vi "cinitel_stabilizace.vi"() -> ()   [LabVIEW 2024]
uses:
  <vilib>/Analysis/baseanly.llb/Mean (DBL).vi
  <instrlib>/EFmeter/EFmeter.lvlib
  <vilib>/Analysis/NI_AALBase.lvlib
  <instrlib>/Zatez Kopper/Zatez Kopper.lvlib
panel:
  in  "Typ zateze":u16(ring) items=["Manualni", "BK 8542B", "Zatez Kopper"]
  in  "VISA EFmeter":refnum<visa-resource-name>
  out "R_out":dbl
  in  "file path (use dialog)":path
  in  "Prodleva mezi vzorky":u32
  out "Aktualni zatez":dbl=2.5
  in  "velikost kroku":dbl
  in  "start":dbl
  in  "Prumerovani":bool
  in  "Vzorku na krokù":u16 max=100 step=1
  out "XY Graph 2":cluster{"X":dbl[], "Y":dbl[]}[](graph)
  in  "Pocet kroku":i32
  in  "Clear":bool
  in  "Uložit data":bool
  in  "Start":bool
  in  "VISA  zatez":refnum<visa-resource-name>
  in  "stop":bool
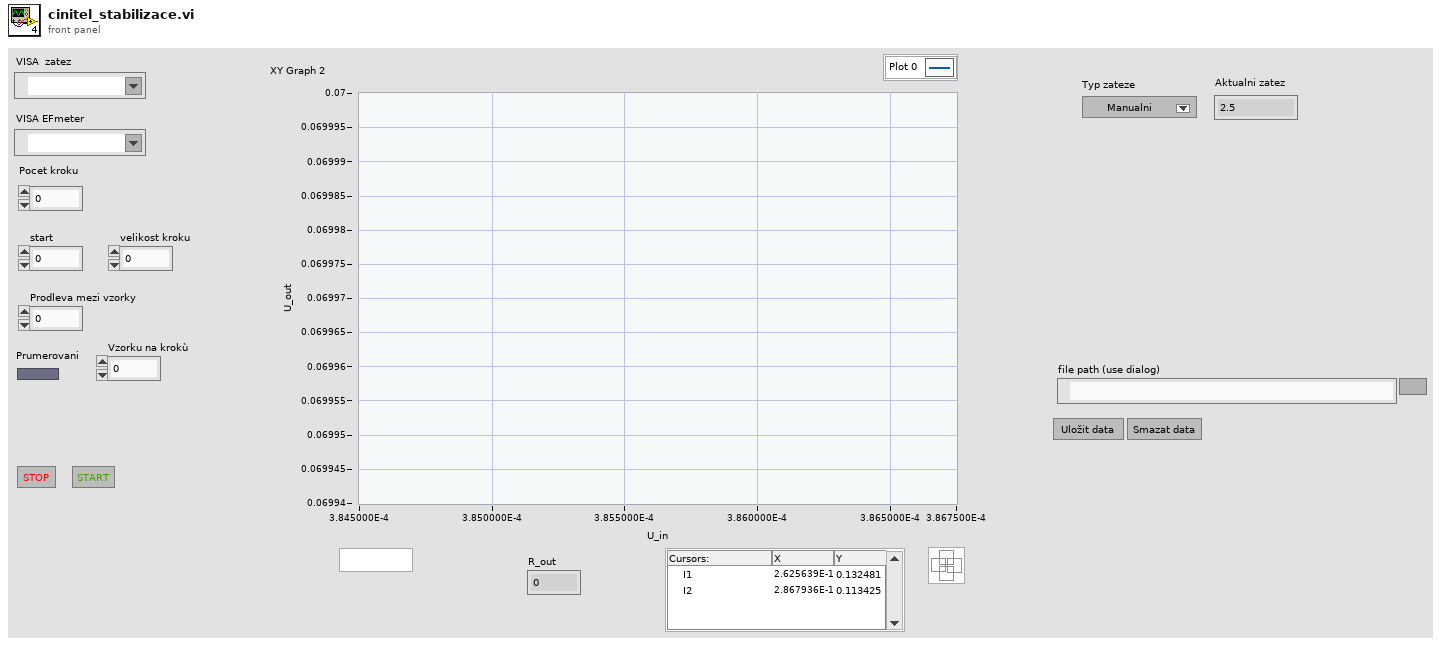
[diagram p1: front panel]
types:
  T1 = enum16{"init", "wait", "graph", "meas", "change_load", "init_measurment", "save", "clear"}
  T2 = typedef "LVCursorListTypeDef.ctl" = cluster{"Name":string, "Color":u32, "Style":u8, "Point Style":u8, "Name Visible":bool, "Allow Drag":bool, "Cursor Mode":u32, "Plot":i32, "Index":i32, "Position":cluster{"X":dbl, "Y":dbl}, "X Scale":u32, "Y Scale":u32, "Watch Plots":i32[], "Watch All Plots":bool, "Plot Area":i32, "Label Offset":cluster{"X":dbl, "Y":dbl}}[]
  T3 = cluster{"Name":string, "Color":u32, "Style":u8, "Point Style":u8, "Name Visible":bool, "Allow Drag":bool, "Cursor Mode":u32, "Plot":i32, "Index":i32, "Position":cluster{"X":dbl, "Y":dbl}, "X Scale":u32, "Y Scale":u32, "Watch Plots":i32[], "Watch All Plots":bool, "Plot Area":i32, "Label Offset":cluster{"X":dbl, "Y":dbl}}
  T4 = enum16{"open", "replace", "create", "open or create", "replace or create", "replace or create with confirmation"}
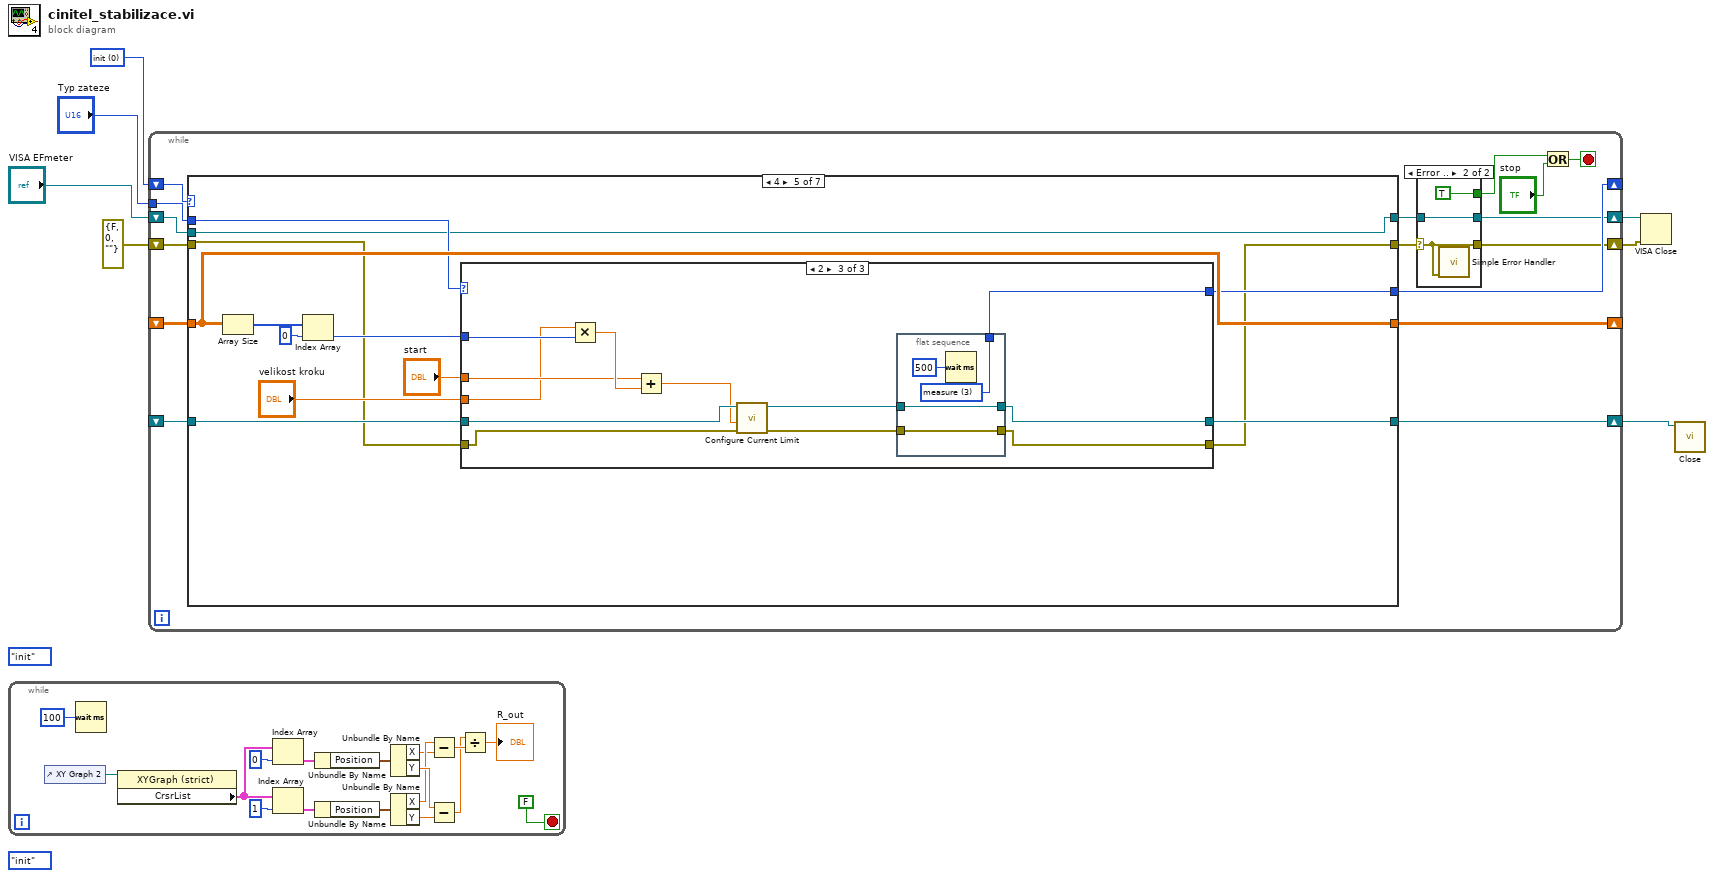
[diagram p0: block diagram]
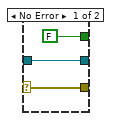
[diagram p2: hidden frame]
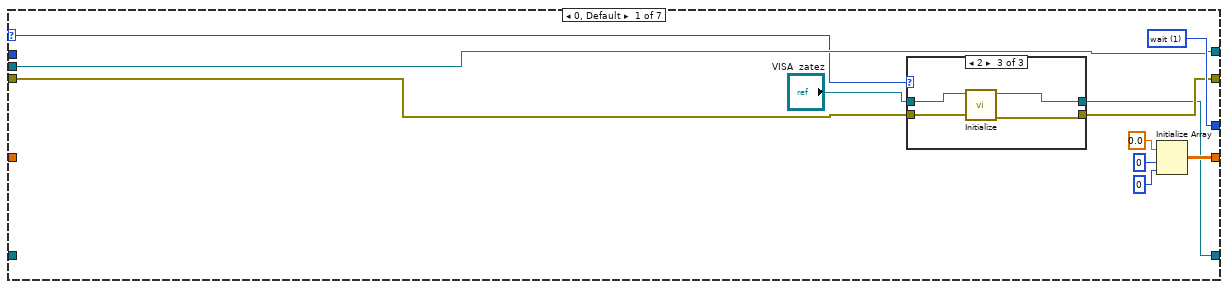
[diagram p3: hidden frame]
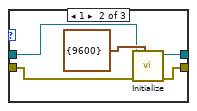
[diagram p5: hidden frame]
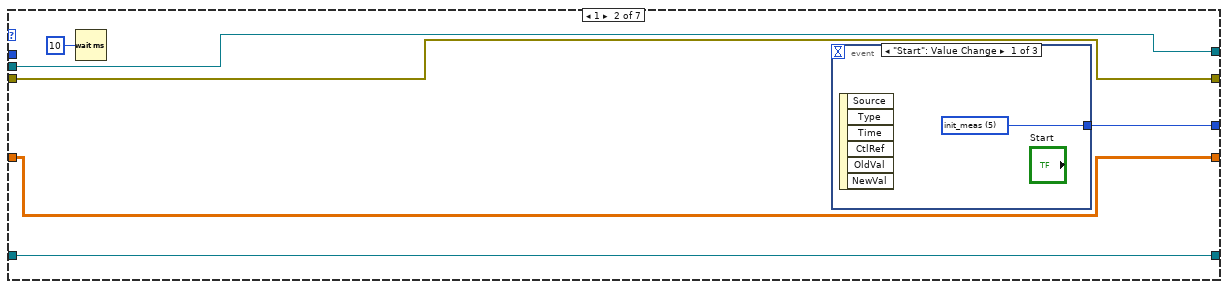
[diagram p6: hidden frame]
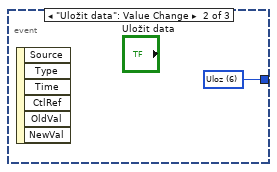
[diagram p7: hidden frame]
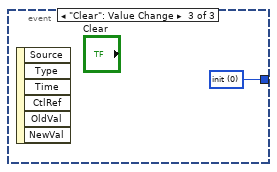
[diagram p8: hidden frame]
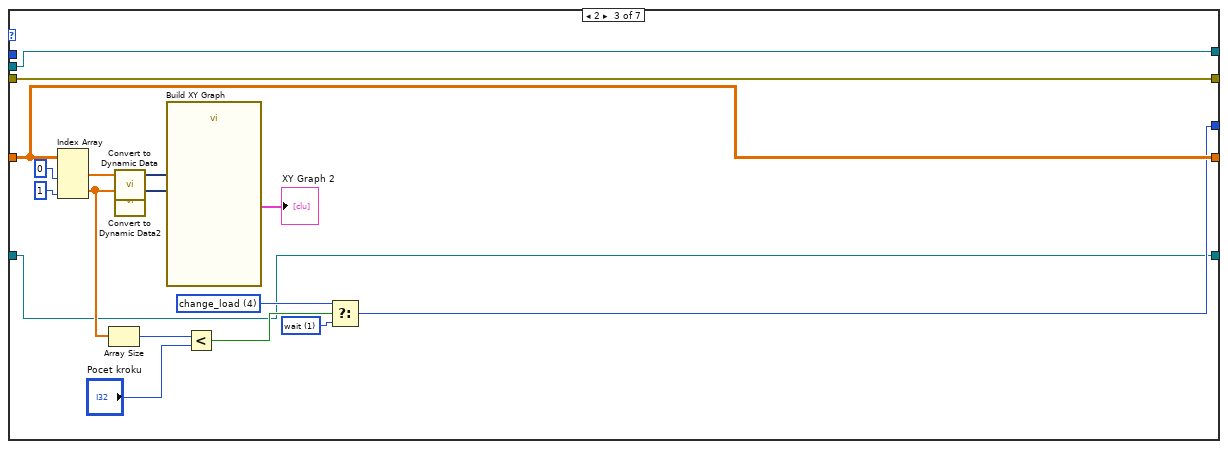
[diagram p9: hidden frame]
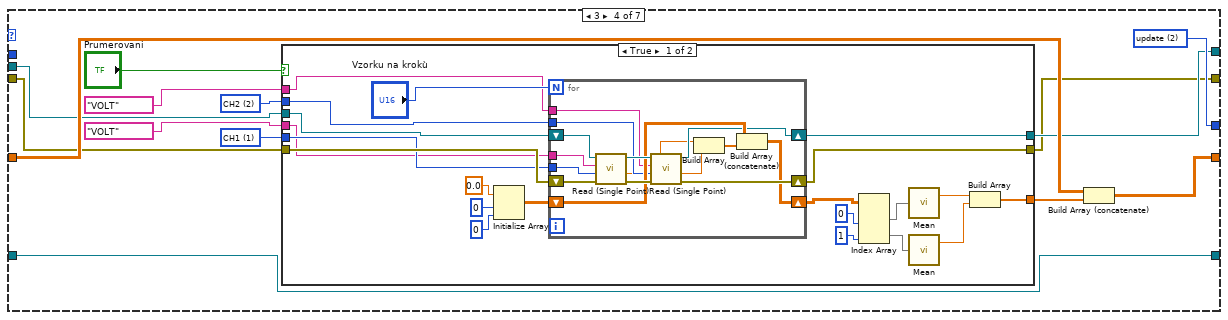
[diagram p10: hidden frame]
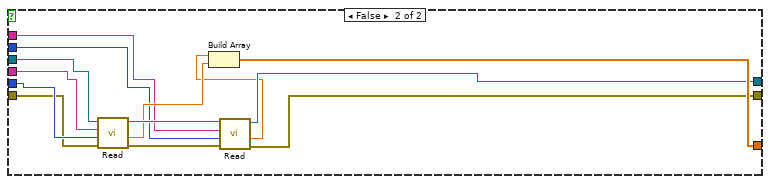
[diagram p11: hidden frame]
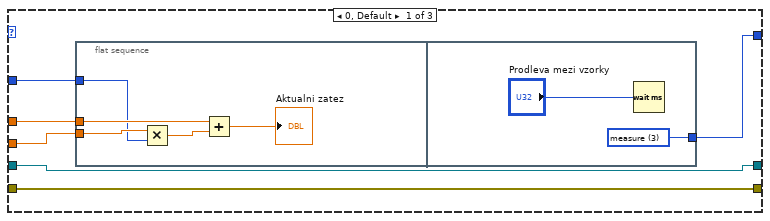
[diagram p12: hidden frame]
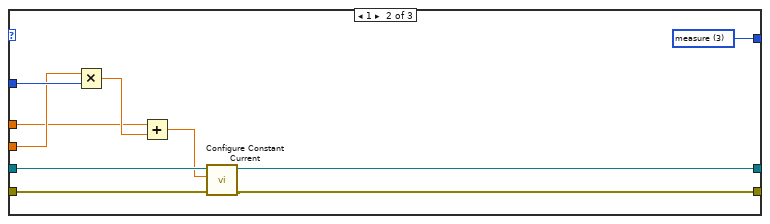
[diagram p13: hidden frame]
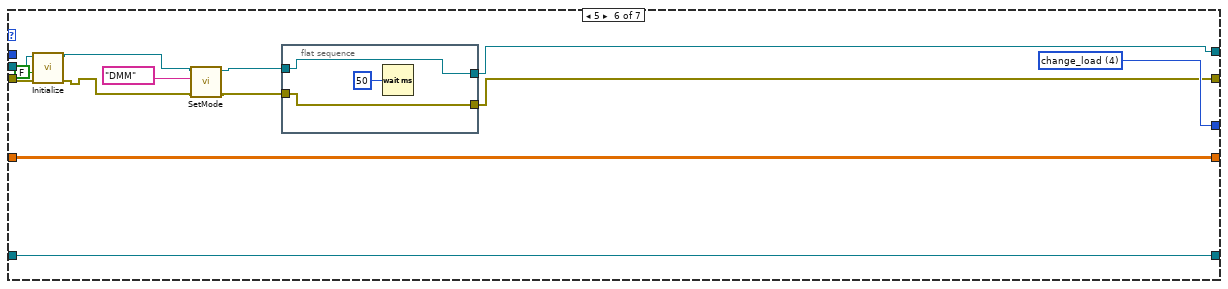
[diagram p14: hidden frame]
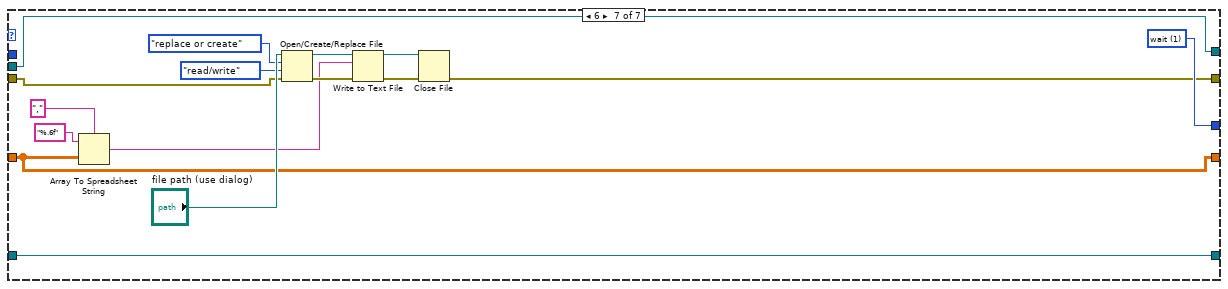
[diagram p15: hidden frame]
diagram:
  (unwired) T1."init"
  (unwired) T1."init"
  w7 = u16 0 items=["init", "wait", "update", "measure", "change_load", "init_meas", "Uloz", "clear"]
  n1 = while {
    stop <- FALSE stop-if-true
    n2 = control-ref of="XY Graph 2"() -> (w22:refnum<vi>)
    n3 = Wait (ms)(milliseconds to wait=u32 100) -> ()  [unwired: 1 out]
    n4 = property class="XYGraph (strict)"(reference=w22) -> ("CrsrList"=w17:T2)  [unwired: 1 in, 2 out]
    n5 = Index Array(array=w17, index=0) -> (element=w23:T3)
    n6 = Index Array(array=w17, index=1) -> (element=w19:T3)
    n7 = Unbundle By Name(w23) -> ("Position"=w24:cluster{"X":dbl, "Y":dbl})
    n8 = Unbundle By Name(w19) -> ("Position"=w20:cluster{"X":dbl, "Y":dbl})
    n9 = Unbundle By Name(w24) -> ("X"=w8:dbl, "Y"=w15:dbl)
    n10 = Unbundle By Name(w20) -> ("X"=w9:dbl, "Y"=w16:dbl)
    n11 = Subtract(x=w9, y=w8) -> (x-y=w11:dbl)
    n12 = Subtract(x=w15, y=w16) -> (x-y=w10:dbl)
    n13 = Divide(x=w10, y=w11) -> (x/y=→"R_out":dbl)
  }
  n14 = while {
    shift-right: [w40] -> _
    shift-left: _ -> [w39]
    shift-right: [w35] -> _
    shift-left: w7 -> [w38]
    shift-right: [w32] -> w4
    shift-left: "VISA EFmeter" -> [w37]
    shift-right: [w25] -> w3
    shift-left: errorcluster {"status"=FALSE, "code"=0, "source"=""} ("error in (no error)") -> [w36]
    tunnel: "Typ zateze" -> [w28]
    shift-right: [w27] -> w1
    shift-left: _ -> [w26]
    stop <- w30 stop-if-true
    n15 = case shown="4" w38 {
      selector: w38 -> [w51 _ _ _ _ _ _]
      tunnel: [w55 w73 w86 w107 w170 w222 w236] -> w40
      tunnel: w39 -> [_ w73 w86 w108 w170 w222 w236]
      tunnel: [w54 w74 w85 w105 w168 w221 w234] -> w35
      tunnel: [w49 w71 w79 w97 w158 w219 w230] -> w34
      tunnel: [w52 w72 w80 w98 w167 w220 w241] -> w33
      tunnel: w37 -> [w52 w72 w80 w104 w167 w217 w241]
      tunnel: w36 -> [w50 w71 w79 w103 w159 w216 w237]
      tunnel: w28 -> [_ _ _ _ w169 _ _]
      tunnel: [w48 w69 w78 w95 w165 w218 w226] -> w27
      tunnel: w26 -> [_ w69 w78 w95 w166 w218 w226]
      frame 0, Default {
        w54 = u16 1 items=["init", "wait", "update", "measure"]
        n16 = case shown="2" w51 {
          tunnel: w50 -> [w59 w63 w68]
          tunnel: [w59 w62 w65] -> w49
          tunnel: [w58 w61 w66] -> w48
          tunnel: "VISA  zatez" -> [w58 w60 w67]
          frame 0, Default {
          }
          frame 1 {
            n17 = call <instrlib>:"Initialize.vi"("Serial Configuration"=cluster{"Baud Rate":u32} {"Baud Rate"=9600}, "error in (no error)"=w63, "VISA resource name"=w60) -> ("error out"=w62:errorcluster, "VISA resource name out"=w61:refnum<visa-resource-name>)  [unwired: 7 in]
          }
          frame 2 {
            n18 = call <instrlib>:"Initialize.vi"("error in (no error)"=w68, "VISA resource name"=w67) -> ("error out"=w65:errorcluster, "VISA resource name out"=w66:refnum<visa-resource-name>)  [unwired: 8 in]
          }
        }
        n19 = Initialize Array(0.0 ("element"), 0 ("dimension size"), 0 ("dimension size")) -> (w55:dbl[][])
      }
      frame 1 {
        n20 = Wait (ms)(milliseconds to wait=u32 10) -> ()  [unwired: 1 out]
        n21 = event shown="[0] \"Start\": Value Change" {
          selector: _ -> [_ _ _]
          dyn-events: _ -> [_ _ _]
          timeout: _ -> [_ _ _]
          tunnel: [w75 w76 w77] -> w74
          event "Start": Value Change {
            w75 = u16 5 items=["init", "wait", "update", "measure", "change_load", "init_meas"]
            n22 = event-data() -> ()  [unwired: 1 in, 6 out]
          }
          event "Uložit data": Value Change {
            w76 = u16 6 items=["init", "wait", "update", "measure", "change_load", "init_meas", "Uloz"]
            n23 = event-data() -> ()  [unwired: 1 in, 6 out]
          }
          event "Clear": Value Change {
            w77 = u16 0 items=["init", "wait", "update", "measure", "change_load", "init_meas", "Uloz", "clear"]
            n24 = event-data() -> ()  [unwired: 1 in, 6 out]
          }
        }
      }
      frame 2 {
        w81 = u16 4 items=["init", "wait", "update", "measure", "change_load", "init_meas"]
        w87 = u16 1 items=["init", "wait", "update", "measure"]
        n25 = Index Array(array=w86, index (col) #1=0 ("index (row)"), index (col) #2=1 ("index (row)")) -> (element #1=w94:dbl[], element #2=w89:dbl[])  [unwired: 2 in]
        n26 = Array Size(array=w89) -> (size(s)=w91:i32)
        n27 = call "Convert to Dynamic Data"("Array"=w94) -> ("Dynamic Data Type"=w93:dynamicdata)  [unwired: 3 in]
        n28 = call "Convert to Dynamic Data2"("Array"=w89) -> ("Dynamic Data Type"=w92:dynamicdata)  [unwired: 3 in]
        n29 = call "Build XY Graph"("Y Input"=w92, "X Input"=w93) -> ("XY Graph"=→"XY Graph 2":cluster{"X":dbl[], "Y":dbl[]}[])  [unwired: 8 in, 1 out]
        n30 = Less?(x=w91, y="Pocet kroku") -> (x < y?=w90:bool)
        n31 = Select(t=w81, s=w90, f=w87) -> (s? t:f=w85:u16)
      }
      frame 3 {
        w99 = u16 2 items=["CH2"=2, "CH1"=1] ("Ring")
        w102 = u16 1 items=["CH2"=2, "CH1"=1] ("Ring")
        w105 = u16 2 items=["init", "wait", "update", "measure"]
        n32 = case shown="True" "Prumerovani" {
          tunnel: [w111 w157] -> w106
          tunnel: w104 -> [w124 w156]
          tunnel: w103 -> [w123 w153]
          tunnel: w102 -> [w122 w154]
          tunnel: "VOLT" ("Combo Box") -> [w121 w155]
          tunnel: "VOLT" ("Combo Box") -> [w120 w149]
          tunnel: w99 -> [w119 w148]
          tunnel: [w110 w147] -> w98
          tunnel: [w109 w146] -> w97
          frame True {
            n33 = Initialize Array(0.0 ("element"), 0 ("dimension size"), 0 ("dimension size")) -> (w125:dbl[][])
            n34 = for {
              N: "Vzorku na krokù" -> [_]
              shift-right: [w140] -> w110
              shift-left: w124 -> [w141]
              shift-right: [w138] -> w109
              shift-left: w123 -> [w139]
              tunnel: w122 -> [w137]
              tunnel: w121 -> [w136]
              tunnel: w120 -> [w135]
              tunnel: w119 -> [w134]
              shift-right: [w133] -> w118
              shift-left: w125 -> [w142]
              n35 = call <instrlib>:"Read (Single Point).vi"("error in (no error)"=w139, "Ring"=w137, "Combo Box"=w136, "VISA resource name"=w141) -> ("error out"=w143:errorcluster, "Measurement"=w131:dbl, "VISA resource name out"=w144:refnum<visa-resource-name>)  [unwired: 5 in]
              n36 = call <instrlib>:"Read (Single Point).vi"("error in (no error)"=w143, "Ring"=w134, "Combo Box"=w135, "VISA resource name"=w144) -> ("error out"=w138:errorcluster, "Measurement"=w132:dbl, "VISA resource name out"=w140:refnum<visa-resource-name>)  [unwired: 5 in]
              n37 = Build Array(w131, w132) -> (w130:dbl[])
              n38 = Build Array (concatenate)(w142, w130) -> (w133:dbl[][])
            }
            n39 = Index Array(array=w118, index (col) #1=0 ("disabled index (col)"), index (col) #2=1 ("index (col)")) -> (element #1=w117:dbl[], element #2=w116:dbl[])  [unwired: 2 in]
            n40 = call-poly <vilib>:"Mean.vi"("X"=w117) -> ("mean"=w113:dbl)  [unwired: 1 out]
            n41 = call-poly <vilib>:"Mean.vi"("X"=w116) -> ("mean"=w112:dbl)  [unwired: 1 out]
            n42 = Build Array(w113, w112) -> (w111:dbl[])
          }
          frame False {
            n43 = call-poly <instrlib>:"Read.vi"("error in (no error)"=w153, "Ring"=w154, "Combo Box"=w155, "VISA resource name"=w156) -> ("error out"=w151:errorcluster, "Measurement"=w150:dbl, "VISA resource name out"=w152:refnum<visa-resource-name>)  [unwired: 5 in]
            n44 = call-poly <instrlib>:"Read.vi"("error in (no error)"=w151, "Ring"=w148, "Combo Box"=w149, "VISA resource name"=w152) -> ("error out"=w146:errorcluster, "Measurement"=w145:dbl, "VISA resource name out"=w147:refnum<visa-resource-name>)  [unwired: 5 in]
            n45 = Build Array(w145, w150) -> (w157:dbl[])
          }
        }
        n46 = Build Array (concatenate)(w108, w106) -> (w107:dbl[][])
      }
      frame 4 {
        n47 = Array Size(array=w170) -> (size(s)=w160:i32[])
        n48 = Index Array(array=w160, index=0) -> (element=w162:i32)
        n49 = case shown="2" w169 {
          tunnel: [w176 w193 w194] -> w168
          tunnel: w166 -> [w175 w192 w200]
          tunnel: [w175 w191 w195] -> w165
          tunnel: "velikost kroku" -> [w174 w189 w202]
          tunnel: "start" -> [w173 w187 w203]
          tunnel: w162 -> [w172 w190 w204]
          tunnel: w159 -> [w171 w185 w201]
          tunnel: [w171 w184 w197] -> w158
          frame 0, Default {
            n50 = flat-sequence {
              tunnel: w174 -> [w179]
              tunnel: w173 -> [w178]
              tunnel: w172 -> [w177]
              tunnel: [w182] -> w176
              frame #0 {
                n51 = Multiply(x=w179, y=w177) -> (x*y=w181:dbl)
                n52 = Add(x=w178, y=w181) -> (x+y=→"Aktualni zatez":dbl)
              }
              frame #1 {
                w182 = u16 3 items=["init", "wait", "update", "measure", "change_load", "init_meas"]
                n53 = Wait (ms)(milliseconds to wait="Prodleva mezi vzorky") -> ()  [unwired: 1 out]
              }
            }
          }
          frame 1 {
            w193 = u16 3 items=["init", "wait", "update", "measure", "change_load", "init_meas"]
            n54 = Multiply(x=w189, y=w190) -> (x*y=w188:dbl)
            n55 = Add(x=w187, y=w188) -> (x+y=w186:dbl)
            n56 = call "Configure Constant Current.vi"("error in (no error)"=w185, "CC Current (0)"=w186, "VISA resource name"=w192) -> ("error out"=w184:errorcluster, "VISA resource name out"=w191:refnum<visa-resource-name>)  [unwired: 7 in]
          }
          frame 2 {
            n57 = Multiply(x=w202, y=w204) -> (x*y=w205:dbl)
            n58 = Add(x=w203, y=w205) -> (x+y=w199:dbl)
            n59 = call <instrlib>:"Configure Current Limit.vi"("error in (no error)"=w201, "Current Limit (0.0 A)"=w199, "VISA resource name"=w200) -> ("error out"=w198:errorcluster, "VISA resource name out"=w196:refnum<visa-resource-name>)  [unwired: 7 in]
            n60 = flat-sequence {
              tunnel: w198 -> [w209]
              tunnel: [w209] -> w197
              tunnel: [w208] -> w195
              tunnel: w196 -> [w208]
              tunnel: [w207] -> w194
              frame #0 {
                w207 = u16 3 items=["init", "wait", "update", "measure", "change_load", "init_meas", "Uloz", "clear"]
                n61 = Wait (ms)(milliseconds to wait=u32 500) -> ()  [unwired: 1 out]
              }
            }
          }
        }
      }
      frame 5 {
        w221 = u16 4 items=["init", "wait", "update", "measure", "change_load", "init_meas"]
        n62 = call <instrlib>:"Initialize.vi"("error in (no error)"=w216, "Reset (True)"=FALSE, "VISA resource name"=w217) -> ("error out"=w213:errorcluster, "VISA resource name out"=w214:refnum<visa-resource-name>)  [unwired: 7 in]
        n63 = call <instrlib>:"SetMode.vi"("error in (no error)"=w213, "Combo Box"="DMM", "VISA resource name"=w214) -> ("error out"=w212:errorcluster, "VISA resource name out"=w211:refnum<visa-resource-name>)  [unwired: 7 in]
        n64 = flat-sequence {
          tunnel: [w224] -> w220
          tunnel: w211 -> [w224]
          tunnel: w212 -> [w223]
          tunnel: [w223] -> w219
          frame #0 {
            n65 = Wait (ms)(milliseconds to wait=u32 50) -> ()  [unwired: 1 out]
          }
        }
      }
      frame 6 {
        w234 = u16 1 items=["init", "wait", "update", "measure", "change_load", "init_meas"]
        n66 = Array To Spreadsheet String(delimiter (Tab)=",", array=w236, 3:"%.6f" ("format string")) -> (spreadsheet string=w227:string)
        n67 = Open/Create/Replace File(file path (use dialog)="file path (use dialog)", error in=w237, operation (0:open)=T4."replace or create", access (0:read/write)=enum16{"read/write", "read-only", "write-only"}."read/write") -> (refnum out=w229:refnum<file>, error out=w232:errorcluster)  [unwired: 2 in, 1 out]
        n68 = Write to Text File(file (use dialog)=w229, text=w227, error in=w232) -> (refnum out=w228:refnum<file>, error out=w231:errorcluster)  [unwired: 1 in, 1 out]
        n69 = Close File(refnum=w228, error in=w231) -> (error out=w230:errorcluster)  [unwired: 1 out]
      }
    }
    n70 = case shown="Error .." w34 {
      selector: w34 -> [w41 w44]
      tunnel: w33 -> [w43 w46]
      tunnel: [w43 w46] -> w32
      tunnel: [w41 w44] -> w25
      tunnel: [FALSE TRUE] -> w29
      frame No Error {
      }
      frame Error {
        n71 = call <vilib>:"Simple Error Handler.vi"("error in (no error)"=w44) -> ()  [unwired: 4 in, 5 out]
      }
    }
    n72 = Or(x=w29, y="stop") -> (x .or. y?=w30:bool)
  }
  n73 = VISA Close(VISA resource name=w4, error in (no error)=w3) -> ()  [unwired: 1 out]
  n74 = call "Close.vi"("VISA resource name"=w1) -> ()  [unwired: 10 in, 1 out]
